vi "Globe Address.vi"(8 "error in (no error)":errorcluster caption="错误输入（无错误）", 10 "Tag":string, 11 "file path (dialog if empty)":path caption="文件路径 （空时为对话框）") -> (0 "error out":errorcluster, 1 "IP":string, 2 "Data Type":T1(ring), 3 "ddress":T2={"Address Areas"=130, "Data Type"=enum."Byte", "DB.No"=0, "Byte"=0, "Length"=0, "Item"=0} {"Address Areas" items=["Input (I)"=129, "Output (Q)"=130, "Bit Memory (M)"=131, "Data (DB)"=132]})   [LabVIEW 2014]
panel:
  out "String":string
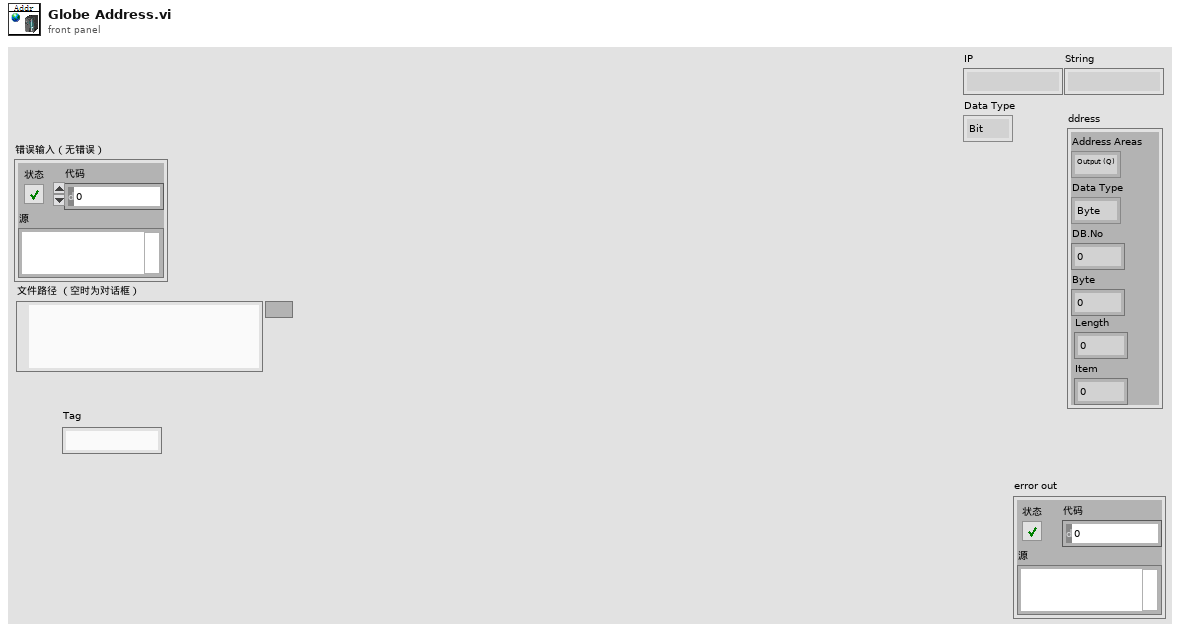
[diagram p1: front panel]
types:
  T1 = enum8{"Bit", "Byte", "int", "Word", "Dint", "Dword", "Real", "String"}
  T2 = typedef "PLC Address.ctl" = cluster{"Address Areas":u8, "Data Type":enum8{"Bit", "Byte", "int", "Word", "Dint", "Dword", "Real", "String"}, "DB.No":u16, "Byte":u32, "Length":u16, "Item":u16}
  T3 = cluster{"ddress":T2, "Data Type":enum8{"Bit", "Byte", "int", "Word", "Dint", "Dword", "Real", "String"}, "IP Address":string}
  T4 = cluster{"Sign Name":string, "IP Address":string, "Type":string, "Target Address":string, "Dir":string, "Remark":string}[]
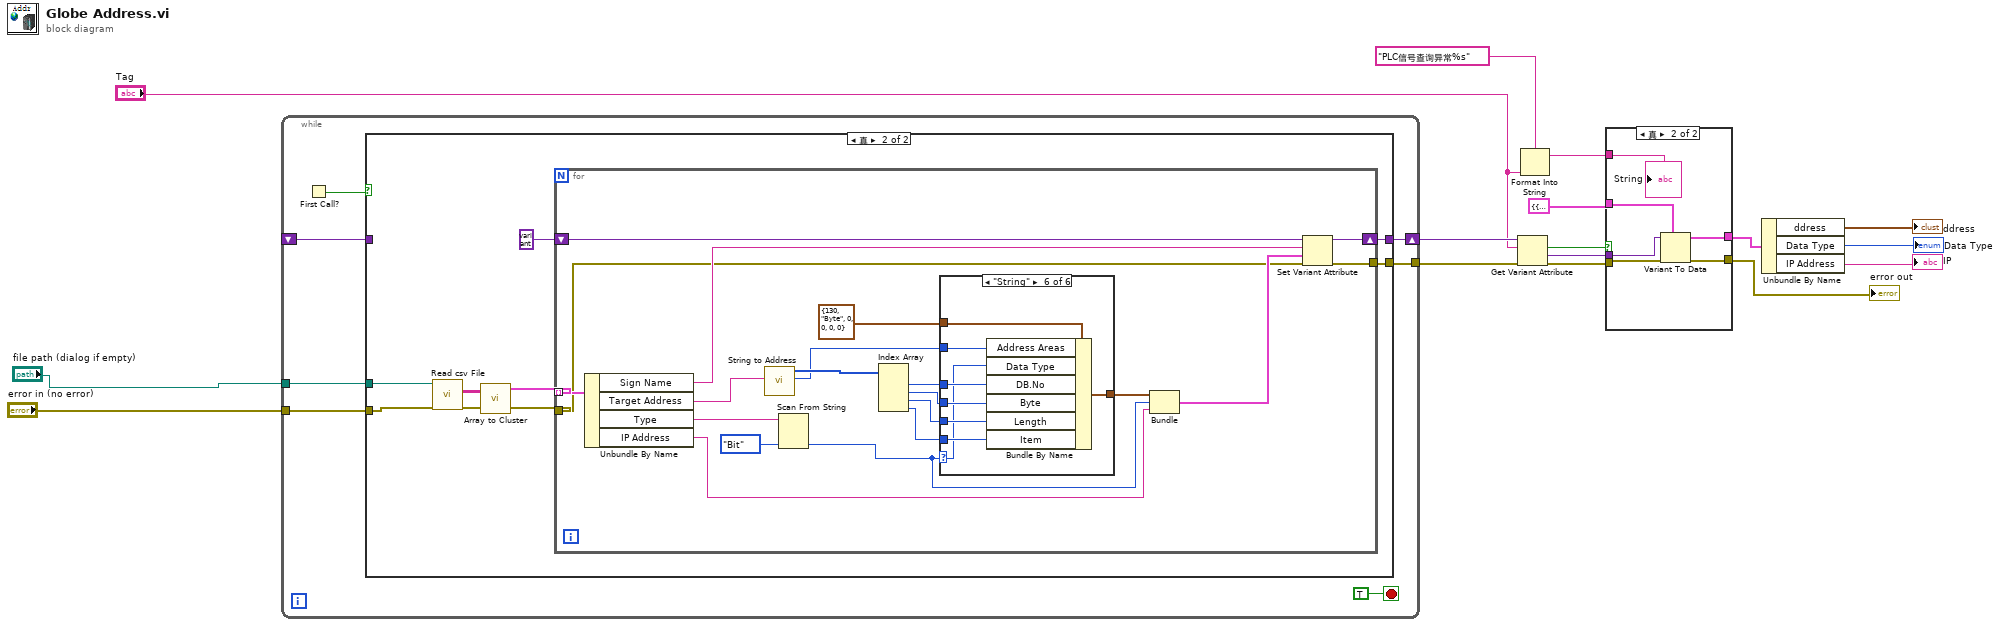
[diagram p0: block diagram]
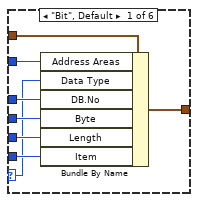
[diagram p4: hidden frame]
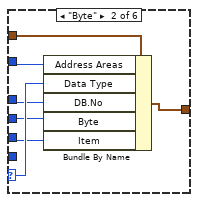
[diagram p5: hidden frame]
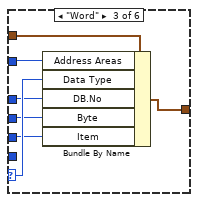
[diagram p6: hidden frame]
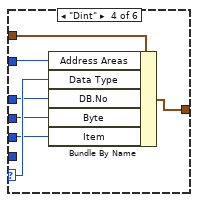
[diagram p7: hidden frame]
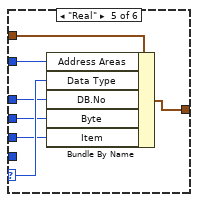
[diagram p8: hidden frame]
diagram:
  n1 = while {
    shift-right: [w22] -> w16
    shift-left: _ -> [w20]
    tunnel: "error in (no error)" -> [w19]
    tunnel: [w18] -> w15
    tunnel: "file path (dialog if empty)" -> [w17]
    stop <- TRUE stop-if-true
    n2 = First Call?() -> (First Call?: T/F=w21:bool)
    n3 = case shown="真" w21 {
      tunnel: [w25 w32] -> w22
      tunnel: w20 -> [w25 _]
      tunnel: w19 -> [w24 w28]
      tunnel: [w24 w31] -> w18
      tunnel: w17 -> [_ w29]
      frame False {
      }
      frame True {
        n4 = call "Read csv File.vi"("error in (no error)"=w28, "file path (dialog if empty)"=w29) -> ("error out"=w27:errorcluster, "all rows"=w30:string[][])  [unwired: 7 in, 1 out]
        n5 = call "Array to Cluster.vi"("2D Array"=w30) -> ("Address"=w26:T4)  [unwired: 4 in]
        n6 = for {
          tunnel: w26 -> [w53] mode=indexing
          shift-right: [w37] -> w32
          shift-left: variant -> [w42]
          tunnel: w27 -> [w36]
          tunnel: [w35] -> w31
          n7 = Unbundle By Name(w53) -> ("Sign Name"=w41:string, "Target Address"=w52:string, "Type"=w51:string, "IP Address"=w34:string)
          n8 = call "String to Address.vi"("Str"=w52) -> ("Type"=w48:u16, "Address"=w50:i32[])  [unwired: 9 in]
          n9 = Scan From String(input string=w51, default 1=T1."Bit" ("Data Type")) -> (output 1=w39:T1)  [unwired: 3 in, 3 out]
          n10 = Index Array(array=w50) -> (element #1=w47:i32, element #2=w46:i32, element #3=w45:i32, element #4=w44:i32)  [unwired: 4 in]
          n11 = case shown="\"String\"" w39 {
            selector: w39 -> [w54 w66 w73 w80 w87 w90]
            tunnel: T2 {"Address Areas"=130, "Data Type"=enum."Byte", "DB.No"=0, "Byte"=0, "Length"=0, "Item"=0} ("ddress") -> [w61 w68 w75 w82 w89 w97]
            tunnel: w48 -> [w60 w67 w74 w81 w88 w96]
            tunnel: w47 -> [w59 w65 w72 w79 w86 w94]
            tunnel: w46 -> [w58 w64 w71 w78 w85 w93]
            tunnel: w45 -> [w57 w63 w70 w77 w84 w92]
            tunnel: w44 -> [w56 _ _ _ _ w91]
            tunnel: [w55 w62 w69 w76 w83 w95] -> w40
            frame "Bit", Default {
              n12 = Bundle By Name(cluster=w61, "Address Areas"=w60, "Data Type"=w54, "DB.No"=w59, "Byte"=w58, "Length"=w57, "Item"=w56) -> (w55:T2)
            }
            frame "Byte" {
              n13 = Bundle By Name(cluster=w68, "Address Areas"=w67, "Data Type"=w66, "DB.No"=w65, "Byte"=w64, "Item"=w63) -> (w62:T2)
            }
            frame "Word" {
              n14 = Bundle By Name(cluster=w75, "Address Areas"=w74, "Data Type"=w73, "DB.No"=w72, "Byte"=w71, "Item"=w70) -> (w69:T2)
            }
            frame "Dint" {
              n15 = Bundle By Name(cluster=w82, "Address Areas"=w81, "Data Type"=w80, "DB.No"=w79, "Byte"=w78, "Item"=w77) -> (w76:T2)
            }
            frame "Real" {
              n16 = Bundle By Name(cluster=w89, "Address Areas"=w88, "Data Type"=w87, "DB.No"=w86, "Byte"=w85, "Item"=w84) -> (w83:T2)
            }
            frame "String" {
              n17 = Bundle By Name(cluster=w97, "Address Areas"=w96, "Data Type"=w90, "DB.No"=w94, "Byte"=w93, "Length"=w92, "Item"=w91) -> (w95:T2)
            }
          }
          n18 = Bundle("ddress"=w40, "Data Type"=w39, "IP Address"=w34) -> (w38:T3)  [unwired: 1 in]
          n19 = Set Variant Attribute(Variant=w42, name=w41, value=w38, error in=w36) -> (Variant out=w37:variant, error out=w35:errorcluster)  [unwired: 1 out]
        }
      }
    }
  }
  n20 = Get Variant Attribute(Variant=w16, name="Tag", error in=w15) -> (found=w14:bool, value=w12:variant, error out=w13:errorcluster)  [unwired: 1 in, 1 out]
  n21 = Format Into String(format string="PLC信号查询异常%s", "Tag") -> (resulting string=w8:string)  [unwired: 2 in, 1 out]
  n22 = case shown="真" w14 {
    tunnel: w13 -> [w98 w105]
    tunnel: w12 -> [_ w104]
    tunnel: T3 {"ddress"={"Address Areas"=0, "Data Type"=enum."Bit", "DB.No"=0, "Byte"=0, "Length"=0, "Item"=0}, "Data Type"=enum."Bit", "IP Address"=""} ("output cluster") -> [w99 w103]
    tunnel: [w99 w102] -> w7
    tunnel: [w98 w101] -> w11
    tunnel: w8 -> [_ w100]
    frame False {
    }
    frame True {
      n23 = Variant To Data(error in=w105, type=w103, Variant=w104) -> (data=w102:T3, error out=w101:errorcluster)
      "String" <- w100
    }
  }
  "error out" <- w11
  n24 = Unbundle By Name(w7) -> ("ddress"=→"ddress":T2, "Data Type"=→"Data Type":T1, "IP Address"=→"IP":string)
